vi "Value to Technique Parameter.vi"(0 "Potentiostat Galvanostat in":refnum<class "Potentiostat Galvanostat.lvclass">, 5 "Parameter Label":string, 7 "Parameter Value":variant, 9 "Parameter Index":i32, 11 "error in (no error)":errorcluster) -> (4 "Potentiostat Galvanostat out":refnum<class "Potentiostat Galvanostat.lvclass">, 8 "Technique Parameter":T1 {"Parameter Type" items=["I32 (Long)", "BOOL (Boolean)", "SGL (Single Precision)"]}, 15 "error out":errorcluster)   [LabVIEW 2018, in "Potentiostat Galvanostat.lvclass"]
doc: "This function tests the communication speed between the library and the selected channel. \nNOTE: This function is for advanced user only."
uses:
  Potentiostat Galvanostat.lvclass
  Controls/Technique Parameter.ctl
  Controls/Parameter Type.ctl
  Controls/Error Codes.ctl
  <vilib>/Utility/Data Type/NI_Data Type.lvlib
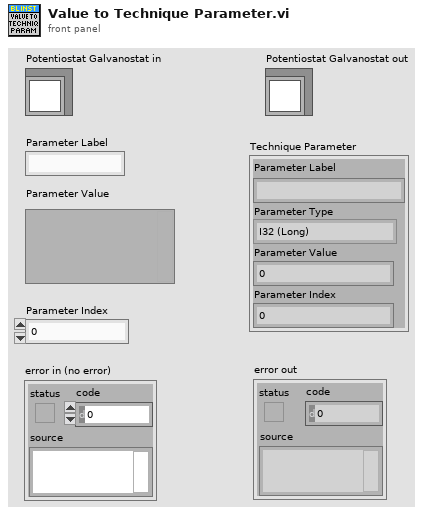
[diagram p1: front panel]
types:
  T1 = typedef "Potentiostat Galvanostat.lvclass/Technique Parameter.ctl" = cluster{"Parameter Label":string, "Parameter Type":T2, "Parameter Value":i32, "Parameter Index":i32}
  T2 = typedef "Potentiostat Galvanostat.lvclass/Parameter Type.ctl" = i32
  T3 = typedef "NI_Data Type.lvlib/Data Type.ctl" = enum8{"Invalid Type", "Void", "I8", "I16", "I32", "I64", "U8", "U16", "U32", "U64", "Single Float", "Double Float", "Extended Float", "Single Complex", "Double Complex", "Extended Complex", "Enum U8", "Enum U16", "Enum U32", "Enum U64", "Single Float With Unit", "Double Float With Unit", "Extended Float With Unit", "Single Complex with Unit", "Double Complex with Unit", "Extended Complex with Unit", "Boolean", "String", "Path", "Picture", "Tag", "Array", "Cluster", "Variant", "LV Variant", "Waveform", "Timestamp", "Digital Waveform", "Digital Data", "ExpressData", "Refnum", "External Data", "VI", "Poly VI", "LabVIEW Class Instance", "Fixed Point"}
  T4 = typedef "Potentiostat Galvanostat.lvclass/Error Codes.ctl" = i32
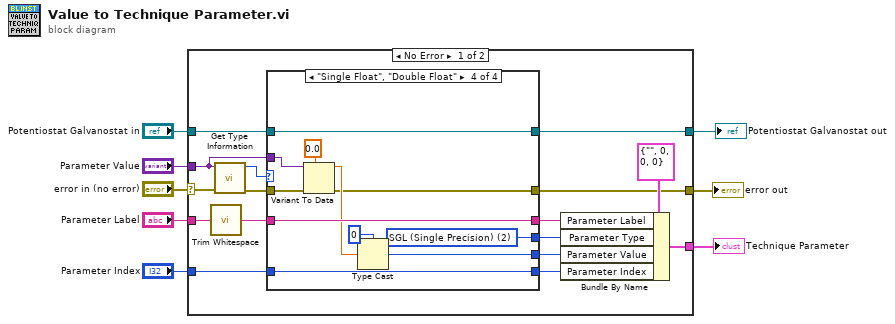
[diagram p0: block diagram]
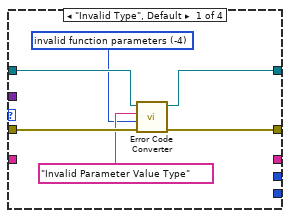
[diagram p2: hidden frame]
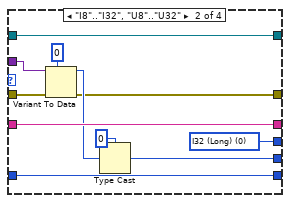
[diagram p3: hidden frame]
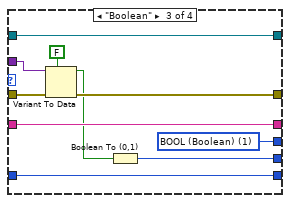
[diagram p4: hidden frame]
diagram:
  n1 = case shown="No Error" "error in (no error)" {
    selector: "error in (no error)" -> [w11 w63]
    tunnel: "Parameter Value" -> [w22 _]
    tunnel: "Potentiostat Galvanostat in" -> [w21 w64]
    tunnel: "Parameter Label" -> [w10 _]
    tunnel: "Parameter Index" -> [w20 _]
    tunnel: [w19 _] -> w4
    tunnel: [w13 w63] -> w3
    tunnel: [w12 w64] -> w2
    frame No Error {
      n2 = call <vilib>:"Trim Whitespace.vi"("string"=w10) -> ("trimmed string"=w9:string)  [unwired: 1 in]
      n3 = call <vilib>:"Get Type Information.vi"("error in (no error)"=w11, "Variant"=w22) -> ("error out"=w23:errorcluster, "Type"=w24:T3)  [unwired: 5 in, 3 out]
      n4 = case shown="\"Single Float\", \"Double Float\"" w24 {
        tunnel: w23 -> [w30 w41 w51 w62]
        tunnel: w22 -> [_ w40 w50 w61]
        tunnel: w21 -> [w29 w31 w44 w52]
        tunnel: [w28 w31 w44 w52] -> w12
        tunnel: [w27 w32 w45 w53] -> w13
        tunnel: w9 -> [_ w38 w48 w59]
        tunnel: w20 -> [_ w37 w47 w58]
        tunnel: [_ w38 w48 w59] -> w17
        tunnel: [_ w33 w46 w54] -> w16
        tunnel: [_ w36 w43 w57] -> w15
        tunnel: [_ w37 w47 w58] -> w14
        frame "Invalid Type", Default {
          w25 = T4 -4 items=["No Error"=0, "no instrument connected"=-1, "connection in progress"=-2, "selected channel(s) unplugged"=-3, "invalid function parameters"=-4, "selected file does not exist"=-5, "function failed"=-6, "no channel selected"=-7, "invalid instrument configuration"=-8, "EC-Lab firmware loaded on the instrument"=-9, "library not correctly loaded in memory"=-10, "USB library not correctly loaded in memory"=-11, "function of the library already in progress"=-12, "selected channel(s) already used"=-13, "device not allowed"=-14, "Invalid update function parameters"=-15, "internal instrument communication failed"=-101, "too many data to transfer from the instrument (device error)"=-102, "selected channel(s) unplugged (device error)"=-103, "instrument response error"=-104, "invalid message size"=-105] ("Error Code")
          n5 = call-dynamic "Error Code Converter.vi"("error in (no error)"=w30, "Error Code"=w25, "Additional Description"="Invalid Parameter Value Type", "Potentiostat Galvanostat in"=w29) -> ("error out"=w27:errorcluster, "Potentiostat Galvanostat out"=w28:refnum<class "Potentiostat Galvanostat.lvclass">)  [unwired: 6 in]
        }
        frame "I8".."I32", "U8".."U32" {
          w33 = T2 0 items=["I32 (Long)", "BOOL (Boolean)", "SGL (Single Precision)"] ("Parameter Type")
          n6 = Variant To Data(error in=w41, type=0, Variant=w40) -> (data=w34:i32, error out=w32:errorcluster)
          n7 = Type Cast(type=0, x=w34) -> (*(type *) &x=w36:i32)
        }
        frame "Boolean" {
          w46 = T2 1 items=["I32 (Long)", "BOOL (Boolean)", "SGL (Single Precision)"] ("Parameter Type")
          n8 = Variant To Data(error in=w51, type=FALSE, Variant=w50) -> (data=w42:bool, error out=w45:errorcluster)
          n9 = Boolean To (0,1)(Boolean=w42) -> (0, 1=w43:i16)
        }
        frame "Single Float", "Double Float" {
          w54 = T2 2 items=["I32 (Long)", "BOOL (Boolean)", "SGL (Single Precision)"] ("Parameter Type")
          n10 = Variant To Data(error in=w62, type=sgl 0.0 ("Numeric"), Variant=w61) -> (data=w55:sgl, error out=w53:errorcluster)
          n11 = Type Cast(type=0, x=w55) -> (*(type *) &x=w57:i32)
        }
      }
      n12 = Bundle By Name(cluster=T1 {"Parameter Label"="", "Parameter Type"=0, "Parameter Value"=0, "Parameter Index"=0} ("Technique Parameter"), "Parameter Label"=w17, "Parameter Type"=w16, "Parameter Value"=w15, "Parameter Index"=w14) -> (w19:T1)
    }
    frame Error {
    }
  }
  "error out" <- w3
  "Potentiostat Galvanostat out" <- w2
  "Technique Parameter" <- w4
